vi "Read Message Class Name.vi"(8 "Error In":errorcluster, 11 "CS++LNAMessage in":refnum<class "CS++LNAMessage.lvclass">) -> (0 "Error Out":errorcluster, 2 "Message Class Name":string, 3 "CS++LNAMessage out":refnum<class "CS++LNAMessage.lvclass">)   [LabVIEW 2014, in "CS++LNA.lvlib" / "CS++LNAMessage.lvclass"]
doc: "Read message class name from attribute."
uses:
  CS++LNAMessage.lvclass
  CS++LNAMessage.lvclass/CS++LNAMessage.ctl
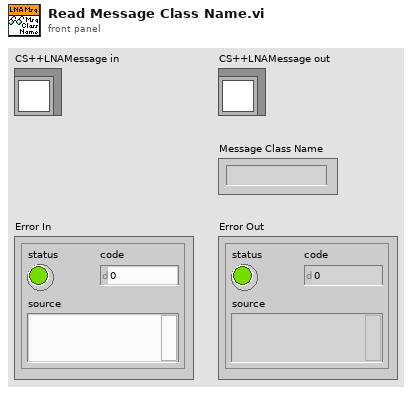
[diagram p1: front panel]
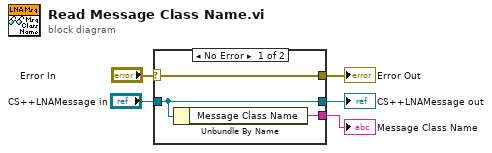
[diagram p0: block diagram]
diagram:
  n1 = case shown="No Error" "Error In" {
    selector: "Error In" -> [w8 w9]
    tunnel: [w8 w9] -> w4
    tunnel: [w7 w10] -> w2
    tunnel: "CS++LNAMessage in" -> [w7 w10]
    tunnel: [w6 _] -> w1
    frame No Error {
      n2 = Unbundle By Name(w7) -> ("Message Class Name"=w6:string)
    }
    frame Error {
    }
  }
  "Error Out" <- w4
  "CS++LNAMessage out" <- w2
  "Message Class Name" <- w1
